vi "Clear Data.vi"(0 "Data In":T1, 1 "Clust Refnum":refnum<vi>, 2 "Time":u32, 3 "error in (no error)":errorcluster) -> (7 "Data Out":T1, 8 "Clust Refnum":refnum<vi>, 10 "error out":errorcluster)   [LabVIEW 2014]
uses:
  controls/Data1.ctl
  controls/Payjson.ctl
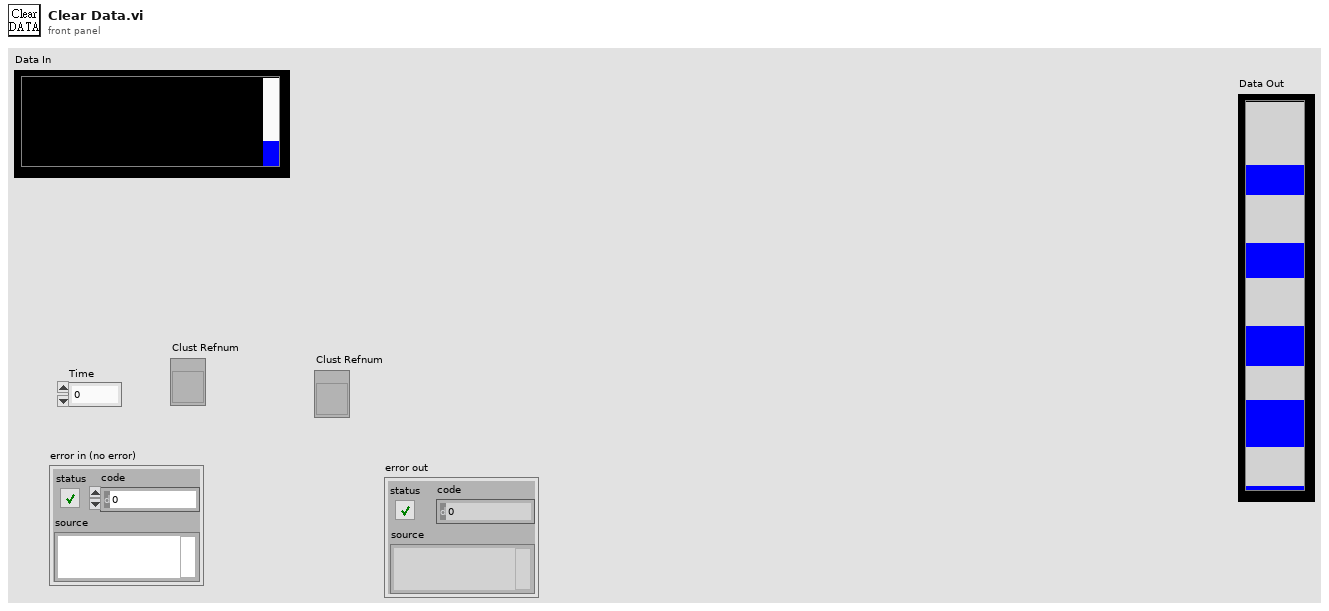
[diagram p1: front panel]
types:
  T1 = typedef "Data1.ctl" = cluster{"Date":string, "BarCode1":string, "BarCode2":string, "BarCode3":string, "Message":string, "OK Count":u16, "NG Count":u16, "Total Count":u16, "ModelData":string[][], "OK&NG":bool, "COM1":refnum<visa-resource-name>, "COM2":refnum<visa-resource-name>, "IO":i32, "Time":u32, "TCP":refnum<k5>, "TCP 2":refnum<k5>, "COM1 2":refnum<visa-resource-name>, "CheckNum":string, "BarCode1_1":string, "BarCode2_1":string, "BarCode3_1":string, "日期":string, "機種":string, "機號":string, "商品條碼1":string, "OK_1":string, "OK":string, "NG":string, "NG_1":string, "Total":string, "Total_1":string, "ClaerTime":u32, "Pjson":T2, "LotNo":string[], "CheckParsArray":string[], "BarCode4":string, "BarCode4_1":string, "商品條碼2":string, "BarCode5":string, "BarCode5_1":string, "商品條碼3":string, "ReScanNG":i32, "NGTimeCT":u32}
  T2 = typedef "Payjson.ctl" = cluster{"DEPT":string, "LINE":string, "STANO":string, "WORKNO":string, "PRODSN":string, "COMPNTID":string, "COMPNTLOT":string, "COMPNTSN":string, "USEDQTY":i16, "OPDATE":string, "OPUSER":string, "RECVDATE":string, "MMODU":string}[]
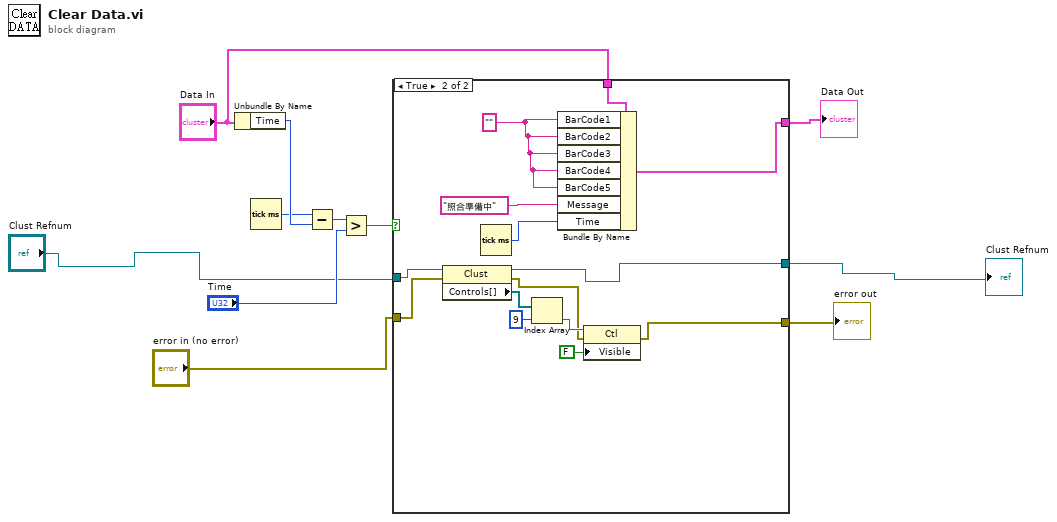
[diagram p0: block diagram]
diagram:
  n1 = Unbundle By Name("Data In") -> ("Time"=w11:u32)
  n2 = Tick Count (ms)() -> (millisecond timer value=w10:u32)
  n3 = Subtract(x=w10, y=w11) -> (x-y=w9:u32)
  n4 = Greater?(x=w9, y="Time") -> (0:w7:bool)
  n5 = case shown="True" w7 {
    tunnel: "Data In" -> [w14 w28]
    tunnel: [w14 w27] -> w5
    tunnel: "error in (no error)" -> [w13 w25]
    tunnel: [w13 w18] -> w3
    tunnel: "Clust Refnum" -> [w12 w26]
    tunnel: [w12 w20] -> w1
    frame False {
    }
    frame True {
      w15 = "" ("BarCode1")
      n6 = property class="Clust"(reference=w26, error in=w25) -> (reference out=w20:refnum<vi>, error out=w21:errorcluster, "Controls[]"=w24:refnum<vi>[])
      n7 = Tick Count (ms)() -> (millisecond timer value=w17:u32)
      n8 = Index Array(array=w24, index=9) -> (element=w22:refnum<vi>)
      n9 = Bundle By Name(cluster=w28, "BarCode1"=w15, "BarCode2"=w15, "BarCode3"=w15, "BarCode4"=w15, "BarCode5"=w15, "Message"="照合準備中", "Time"=w17) -> (w27:T1)
      n10 = property class="Ctl"(reference=w22, error in=w21, "Visible"=FALSE) -> (error out=w18:errorcluster)  [unwired: 1 out]
    }
  }
  "Data Out" <- w5
  "error out" <- w3
  "Clust Refnum" <- w1
